vi "Gather Input.vi"(4 "Shifter":T1, 6 "Gamepad":T1, 8 "Joystick Right":T1, 11 "Joystick Left":T1) -> ()   [LabVIEW 2017]
uses:
  <vilib>/Rock Robotics/WPI/Joystick/WPI_JoystickDevRef.ctl
  <vilib>/Rock Robotics/WPI/Joystick/WPI_JoystickDeviceEnum.ctl
  Joystick Values.vi
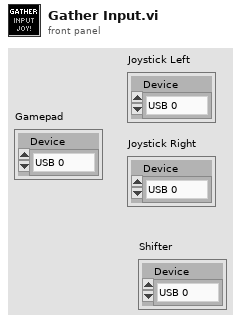
[diagram p1: front panel]
types:
  T1 = typedef "WPI_JoystickDevRef.ctl" = cluster{"Device":T2}
  T2 = typedef "WPI_JoystickDeviceEnum.ctl" = enum16{"USB 0", "USB 1", "USB 2", "USB 3", "USB 4", "USB 5"}
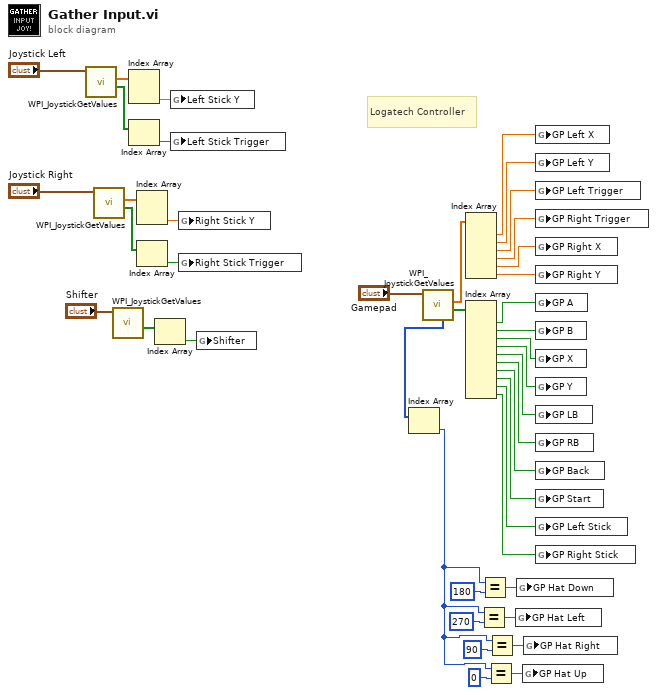
[diagram p0: block diagram]
diagram:
  # "Logatech Controller"
  n1 = call <vilib>:"WPI_JoystickGetValues.vi"("JoystickDevRef"="Joystick Left") -> ("Buttons"=w14:bool[], "Axes"=w13:dbl[])  [unwired: 6 in, 3 out]
  n2 = call <vilib>:"WPI_JoystickGetValues.vi"("JoystickDevRef"="Joystick Right") -> ("Buttons"=w20:bool[], "Axes"=w18:dbl[])  [unwired: 6 in, 3 out]
  n3 = call <vilib>:"WPI_JoystickGetValues.vi"("JoystickDevRef"="Shifter") -> ("Buttons"=w12:bool[])  [unwired: 6 in, 4 out]
  n4 = Index Array(array=w13) -> (element #2=w15:dbl)  [unwired: 2 in, 1 out]
  n5 = Index Array(array=w14) -> (element=w16:bool)  [unwired: 1 in]
  n6 = Index Array(array=w18) -> (element #2=w17:dbl)  [unwired: 2 in, 1 out]
  n7 = Index Array(array=w20) -> (element=w19:bool)  [unwired: 1 in]
  n8 = Index Array(array=w12) -> (element=w11:bool)  [unwired: 1 in]
  n9 = global write "Joystick Values.vi" "Left Stick Y"(w15) -> ()
  n10 = global write "Joystick Values.vi" "Left Stick Trigger"(w16) -> ()
  n11 = global write "Joystick Values.vi" "Right Stick Y"(w17) -> ()
  n12 = global write "Joystick Values.vi" "Right Stick Trigger"(w19) -> ()
  n13 = global write "Joystick Values.vi" "Shifter"(w11) -> ()
  n14 = call <vilib>:"WPI_JoystickGetValues.vi"("JoystickDevRef"="Gamepad") -> ("Buttons"=w41:bool[], "Axes"=w29:dbl[], "POVs"=w9:i16[])  [unwired: 6 in, 2 out]
  n15 = Index Array(array=w9) -> (element=w1:i16)  [unwired: 1 in]
  n16 = Index Array(array=w29) -> (element #1=w30:dbl, element #2=w28:dbl, element #3=w25:dbl, element #4=w24:dbl, element #5=w27:dbl, element #6=w26:dbl)  [unwired: 6 in]
  n17 = Index Array(array=w41) -> (element #1=w40:bool, element #2=w39:bool, element #3=w38:bool, element #4=w37:bool, element #5=w36:bool, element #6=w35:bool, element #7=w34:bool, element #8=w33:bool, element #9=w32:bool, element #10=w31:bool)  [unwired: 10 in]
  n18 = Equal?(x=w1, y=i16 270) -> (x = y?=w6:bool)
  n19 = Equal?(x=w1, y=i16 180) -> (x = y?=w10:bool)
  n20 = Equal?(x=w1, y=i16 0) -> (x = y?=w2:bool)
  n21 = Equal?(x=w1, y=i16 90) -> (x = y?=w3:bool)
  n22 = global write "Joystick Values.vi" "GP Hat Left"(w6) -> ()
  n23 = global write "Joystick Values.vi" "GP Hat Down"(w10) -> ()
  n24 = global write "Joystick Values.vi" "GP Hat Up"(w2) -> ()
  n25 = global write "Joystick Values.vi" "GP Hat Right"(w3) -> ()
  n26 = global write "Joystick Values.vi" "GP Left X"(w30) -> ()
  n27 = global write "Joystick Values.vi" "GP Left Y"(w28) -> ()
  n28 = global write "Joystick Values.vi" "GP Left Trigger"(w25) -> ()
  n29 = global write "Joystick Values.vi" "GP Right Trigger"(w24) -> ()
  n30 = global write "Joystick Values.vi" "GP Right X"(w27) -> ()
  n31 = global write "Joystick Values.vi" "GP Right Y"(w26) -> ()
  n32 = global write "Joystick Values.vi" "GP A"(w40) -> ()
  n33 = global write "Joystick Values.vi" "GP B"(w39) -> ()
  n34 = global write "Joystick Values.vi" "GP X"(w38) -> ()
  n35 = global write "Joystick Values.vi" "GP Y"(w37) -> ()
  n36 = global write "Joystick Values.vi" "GP LB"(w36) -> ()
  n37 = global write "Joystick Values.vi" "GP RB"(w35) -> ()
  n38 = global write "Joystick Values.vi" "GP Back"(w34) -> ()
  n39 = global write "Joystick Values.vi" "GP Start"(w33) -> ()
  n40 = global write "Joystick Values.vi" "GP Left Stick"(w32) -> ()
  n41 = global write "Joystick Values.vi" "GP Right Stick"(w31) -> ()
